vi "Dummy Output.vi"(3 "error in (no error)":errorcluster, 4 "Multi Output":dbl[](array[numeric]) format="%#.2g", 5 "Single Output":dbl format="%#.2g") -> (0 "error out":errorcluster)   [LabVIEW 2023]
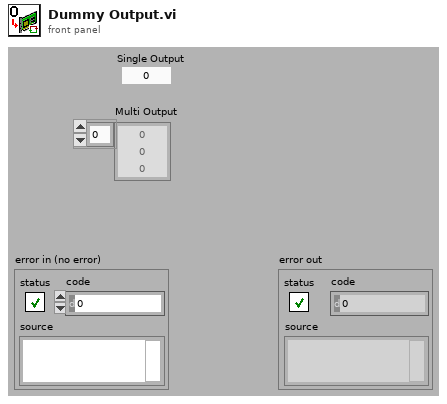
[diagram p1: front panel]
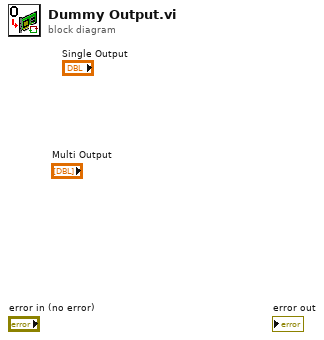
[diagram p0: block diagram]
diagram:
